vi "get Current State.vi"(11 "Clock Generator in":refnum<class "Clock Generator.lvclass">) -> (3 "Current State":bool)   [LabVIEW 2021, in "Clock Generator.lvclass"]
uses:
  Clock Generator.lvclass
  Clock Generator.lvclass/Clock Generator.ctl
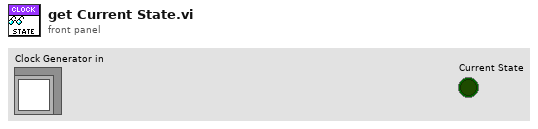
[diagram p1: front panel]
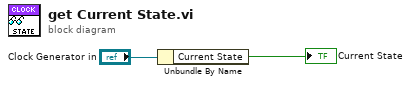
[diagram p0: block diagram]
diagram:
  n1 = Unbundle By Name("Clock Generator in") -> ("Current State"=→"Current State":bool)
